vi "Update Data.vi"(8 "error in (no error)":errorcluster, 9 "data":waveform(dbl)[](array[waveform]), 10 "Channel Names":string[](array[string]), 11 "[V] Main UI in":refnum<class "[V] Main UI.lvclass">) -> (0 "error out":errorcluster, 3 "[V] Main UI out":refnum<class "[V] Main UI.lvclass">)   [LabVIEW 2020, in "[V] Main UI.lvlib" / "[V] Main UI.lvclass"]
uses:
  [V] Main UI.lvclass
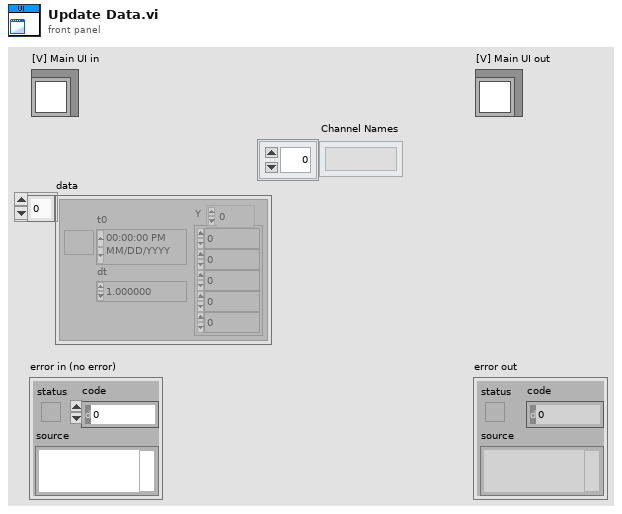
[diagram p1: front panel]
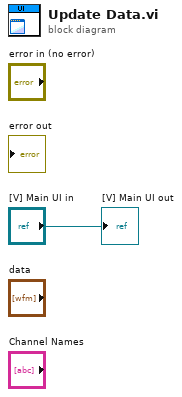
[diagram p0: block diagram]
diagram:
  "[V] Main UI out" <- "[V] Main UI in"
